vi "OE1022D_Operation_Continuous_or_Averaging.vi"() -> ()   [LabVIEW 2024]
uses:
  <vilib>/Utility/file.llb/Write Delimited Spreadsheet (string).vi
  <vilib>/Utility/file.llb/Write Delimited Spreadsheet (DBL).vi
  <vilib>/Analysis/NI_AALBase.lvlib
panel:
  in  "Add file info to file save":bool=TRUE
  in  "B Sensitivity":u16(ring)=20 items=["1 nV/fA", "2 nV/fA", "5 nV/fA", "10 nV/fA", "20 nV/fA", "50 nV/fA", "100 nV/fA", "200 nV/fA", "500 nV/fA", "1 uV/pA", "2 uV/pA", "5 uV/pA", "10 uV/pA", "20 uV/pA", "50 uV/pA", "100 uV/pA", "200 uV/pA", "500 uV/pA", "1 mV/nA", "2 mV/nA", "5 mV/nA", "10 mV/nA", "20 mV/nA", "50 mV/nA", "100 mV/nA", "200 mV/nA", "500 mV/nA", "1 V/uA"]
  out "Channel B Waveform Chart":dbl(graph)
  in  "Channel B Waveform Display":string(combo)="B-R"
  in  "Channel A Waveform Display":string(combo)="A-R"
  in  "A Sensitivity":u16(ring)=20 items=["1 nV/fA", "2 nV/fA", "5 nV/fA", "10 nV/fA", "20 nV/fA", "50 nV/fA", "100 nV/fA", "200 nV/fA", "500 nV/fA", "1 uV/pA", "2 uV/pA", "5 uV/pA", "10 uV/pA", "20 uV/pA", "50 uV/pA", "100 uV/pA", "200 uV/pA", "500 uV/pA", "1 mV/nA", "2 mV/nA", "5 mV/nA", "10 mV/nA", "20 mV/nA", "50 mV/nA", "100 mV/nA", "200 mV/nA", "500 mV/nA", "1 V/uA"]
  in  "File Path":path=path "C:/Users/Public/OneDrive/Desktop/test.txt"
  in  "Data Points":i32
  out "Channel AWaveform Chart":dbl(graph)
  out "θh1 (°) 2":sgl caption="θh1 (deg)" format="%.2f"
  out "Rh1 2":sgl caption="Rh1 (Vrms)" format="%.3p"
  out "Yh1 2":sgl caption="Yh1 (Vrms)" format="%.3p"
  out "Xh1 2":sgl caption="Xh1 (Vrms)" format="%.3p"
  out "Xh2 2":sgl caption="Xh2 (Vrms)" format="%.3p"
  out "Yh2 2":sgl caption="Yh2 (Vrms)" format="%.3p"
  out "Rh2 2":sgl caption="Rh2 (Vrms)" format="%.3p"
  out "噪声 2":sgl caption="Noise(Vrms)" format="%.3p"
  out "频率 (Hz) 2":sgl caption="Freq (Hz)" format="%#.3f"
  out "θ (°) 2":sgl caption="θ (deg)" format="%.2f"
  out "R 2":sgl caption="R (Vrms)" format="%.3p"
  out "Y 2":sgl caption="Y (Vrms)" format="%.3p"
  out "θh2 (°) 2":sgl caption="θh2 (deg)" format="%.2f"
  out "X 2":sgl caption="X (Vrms)" format="%.3p"
  out "Yh1":sgl caption="Yh1 (Vrms)" format="%.3p"
  out "Xh1":sgl caption="Xh1 (Vrms)" format="%.3p"
  out "θh2 (°)":sgl caption="θh2 (deg)" format="%.2f"
  out "Yh2":sgl caption="Yh2 (Vrms)" format="%.3p"
  out "Xh2":sgl caption="Xh2 (Vrms)" format="%.3p"
  out "Rh2":sgl caption="Rh2 (Vrms)" format="%.3p"
  out "θh1 (°)":sgl caption="θh1 (deg)" format="%.2f"
  out "Rh1":sgl caption="Rh1 (Vrms)" format="%.3p"
  out "噪声":sgl caption="Noise(Vrms)" format="%.3p"
  out "频率 (Hz)":sgl caption="Freq (Hz)" format="%#.3f"
  out "θ (°)":sgl caption="θ (deg)" format="%.2f"
  out "Y":sgl caption="Y (Vrms)" format="%.3p"
  out "X":sgl caption="X (Vrms)" format="%.3p"
  out "R":sgl caption="R (Vrms)" format="%.3p"
  out "AUX-ADC2 (V)":sgl format="%.3f"
  out "AUX-ADC1 (V)":sgl format="%.3f"
  out "AUX-ADC3 (V)":sgl format="%.3f"
  out "AUX-ADC4 (V)":sgl format="%.3f"
  out "错误输出":errorcluster
  out "序列号":string
  in  "OE1022D":refnum<visa-resource-name>="COM6"
  # "input 0 for continous"
  # "Choose the value to display on the graph. This is the quantity that is saved"
  # "Channel A"
  # "Channel B"
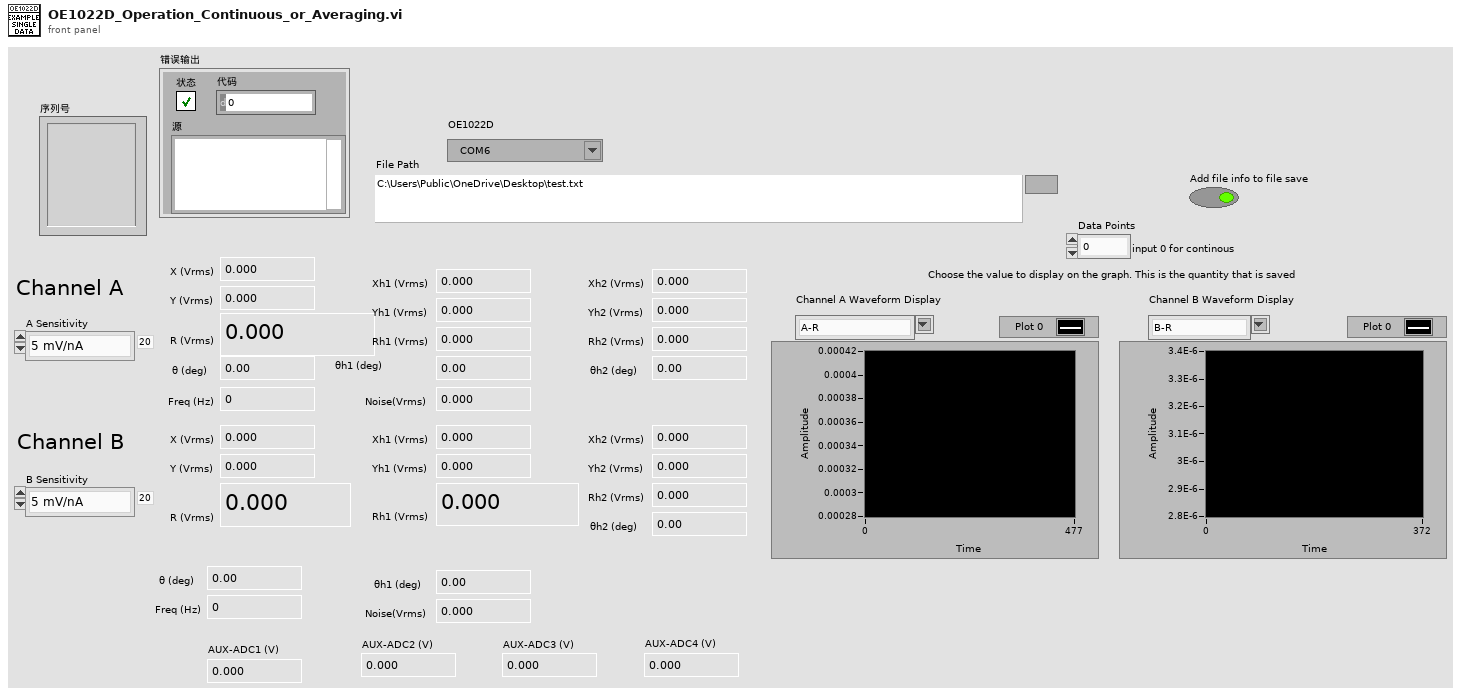
[diagram p1: front panel]
types:
  T1 = cluster{"AD1":dbl[], "AD2":dbl[], "AD3":dbl[], "AD4":dbl[]}
  T2 = cluster{"XB":dbl[], "YB":dbl[], "FrequencyB":dbl[], "NoiseB":dbl[], "Xh1B":dbl[], "Yh1B":dbl[], "Xh2B":dbl[], "Yh2B":dbl[], "Xh2B":dbl[]}
  T3 = cluster{"XA":dbl[], "YA":dbl[], "FrequencyA":dbl[], "NoiseA":dbl[], "Xh1A":dbl[], "Yh1A":dbl[], "Xh2A":dbl[], "Yh2A":dbl[]}
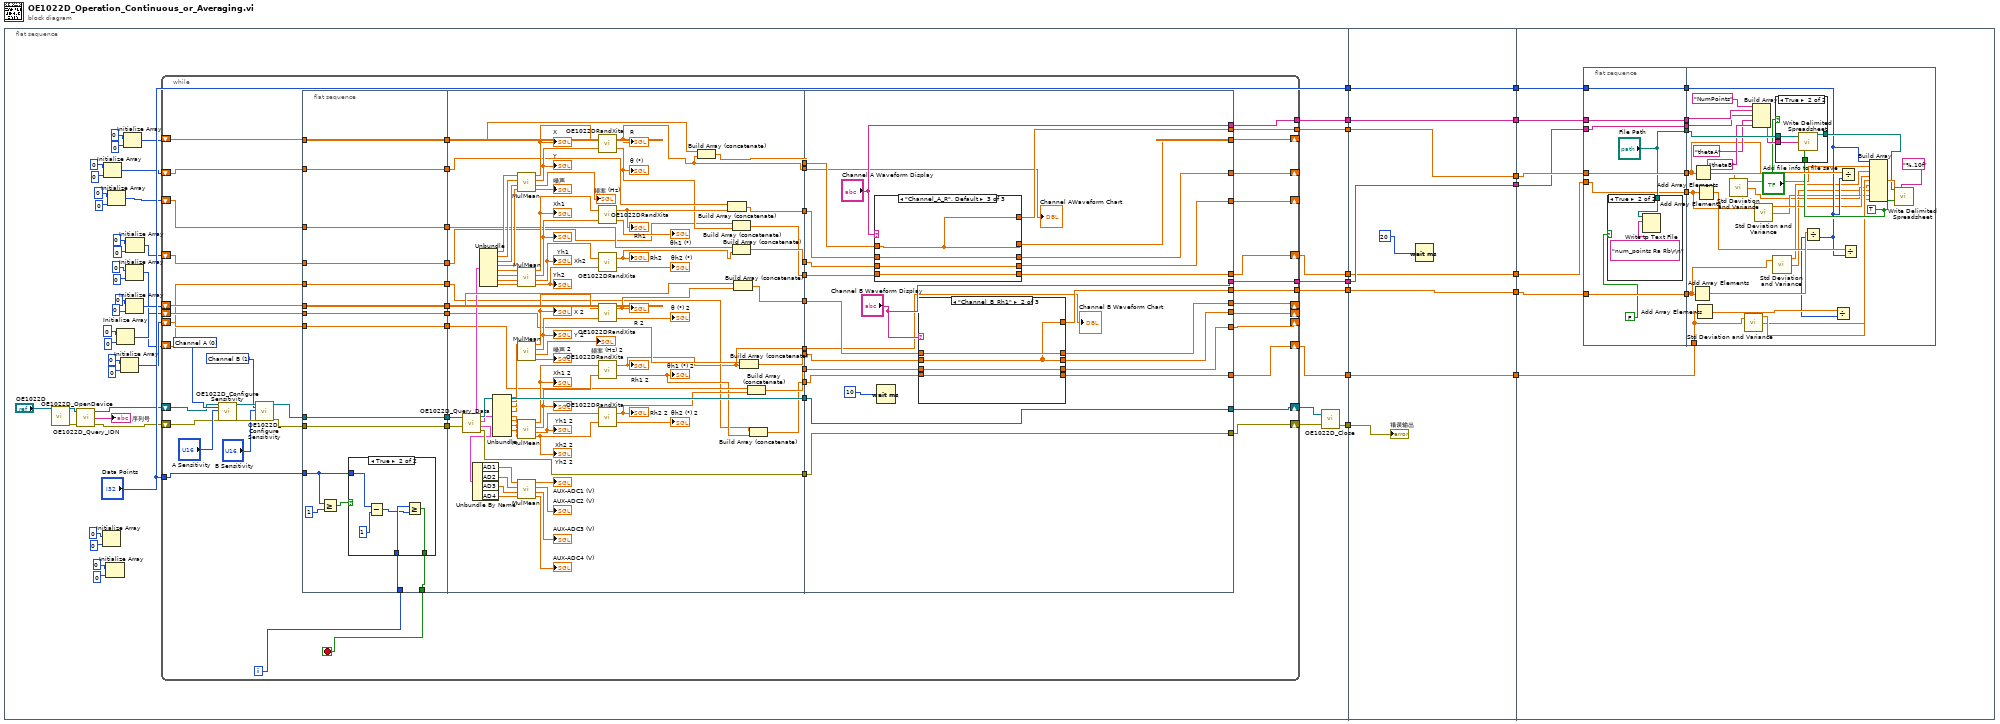
[diagram p0: block diagram]
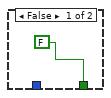
[diagram p2: hidden frame]
diagram:
  n1 = flat-sequence {
    tunnel: [w36] -> w15
    tunnel: [w35] -> w13
    tunnel: ["Data Points"] -> w11
    tunnel: [w30] -> w9
    tunnel: [w34] -> w7
    tunnel: [w33] -> w6
    tunnel: [w20] -> w3
    tunnel: [w21] -> w2
    tunnel: w15 -> [w270]
    tunnel: [w270] -> w14
    tunnel: w13 -> [w269]
    tunnel: [w269] -> w12
    tunnel: w11 -> [w268]
    tunnel: [w268] -> w10
    tunnel: w9 -> [w266]
    tunnel: [w265] -> w8
    tunnel: w7 -> [w265]
    tunnel: w6 -> [w264]
    tunnel: [w264] -> w5
    tunnel: [w263] -> w4
    tunnel: w3 -> [w263]
    tunnel: w2 -> [w262]
    tunnel: [w262] -> w1
    tunnel: w14 -> [w280]
    tunnel: w12 -> [w279]
    tunnel: w10 -> [w278]
    tunnel: w8 -> [w276]
    tunnel: w5 -> [w275]
    tunnel: w4 -> [w273]
    tunnel: w1 -> [w271]
    frame #0 {
      n2 = call "OE1022D_OpenDevice.vi"("VISA resource name"="OE1022D") -> ("VISA资源名称输出"=w58:refnum<visa-resource-name>, "错误输出"=w57:errorcluster)  [unwired: 17 in]
      n3 = call "OE1022D_Query_IDN.vi"("错误输入（无错误）"=w57, "VISA resource name"=w58) -> ("错误输出"=w28:errorcluster, "序列号"=→"序列号":string, "VISA resource name out"=w29:refnum<visa-resource-name>)  [unwired: 1 in]
      n4 = Initialize Array(0, 0) -> ()  [unwired: 1 out]
      n5 = Initialize Array(0, 0) -> (w43:i32[])
      n6 = Initialize Array(0, 0) -> ()  [unwired: 1 out]
      n7 = Initialize Array(0, 0) -> (w44:i32[])
      n8 = Initialize Array(0, 0) -> (w37:i32[])
      n9 = Initialize Array(0, 0) -> (w38:i32[])
      n10 = Initialize Array(0, 0) -> (w54:i32[])
      n11 = Initialize Array(0, 0) -> (w22:i32[])
      n12 = Initialize Array(0, 0) -> (w49:i32[])
      n13 = Initialize Array(0, 0) -> (w23:i32[])
      n14 = while {
        shift-right: [w113] -> _
        shift-left: w54 -> [w112]
        shift-right: [w110] -> _
        shift-left: w49 -> [w109]
        tunnel: "Data Points" -> [w102]
        shift-right: [w90] -> _
        shift-left: w43 -> [w92]
        shift-right: [w86] -> _
        shift-left: w44 -> [w89]
        shift-right: [w79] -> _
        shift-left: w37 -> [w85]
        shift-right: [w78] -> _
        shift-left: w38 -> [w84]
        tunnel: [w77] -> w36
        tunnel: [w76] -> w35
        tunnel: [w75] -> w34
        tunnel: [w74] -> w33
        shift-right: [w73] -> w32
        shift-left: w28 -> [w70]
        shift-right: [w72] -> w31
        shift-left: w29 -> [w71]
        shift-right: [w62] -> w20
        shift-left: w23 -> [w66]
        shift-right: [w63] -> w21
        shift-left: w22 -> [w64]
        i -> [w104]
        stop <- w103 stop-if-true
        w95 = u8 1 items=["Channel A", "Channel B"] ("OE1022D A/B")
        w101 = u8 0 items=["Channel A", "Channel B"] ("OE1022D A/B")
        n15 = call "OE1022D_Configure Sensitivity.vi"("VISA resource name"=w71, "OE1022D A/B"=w101, "Sensitivity"="A Sensitivity", "error in (no error)"=w70) -> ("VISA resource name out"=w96:refnum<visa-resource-name>, "error out"=w97:errorcluster)  [unwired: 14 in]
        n16 = call "OE1022D_Configure Sensitivity.vi"("VISA resource name"=w96, "OE1022D A/B"=w95, "Sensitivity"="B Sensitivity", "error in (no error)"=w97) -> ("VISA resource name out"=w99:refnum<visa-resource-name>, "error out"=w98:errorcluster)  [unwired: 14 in]
        n17 = flat-sequence {
          tunnel: w109 -> [w128]
          tunnel: w112 -> [w129]
          tunnel: w99 -> [w130]
          tunnel: w98 -> [w131]
          tunnel: [w131] -> w108
          tunnel: [w130] -> w107
          tunnel: [w129] -> w106
          tunnel: [w128] -> w105
          tunnel: w104 -> [w127]
          tunnel: [w126] -> w103
          tunnel: w102 -> [w124]
          tunnel: [w122] -> w93
          tunnel: w92 -> [w122]
          tunnel: w89 -> [w121]
          tunnel: [w121] -> w88
          tunnel: w85 -> [w120]
          tunnel: w84 -> [w119]
          tunnel: [w120] -> w83
          tunnel: [w119] -> w82
          tunnel: [w118] -> w67
          tunnel: w66 -> [w118]
          tunnel: [w117] -> w65
          tunnel: w64 -> [w117]
          tunnel: [w210] -> w116
          tunnel: [w209] -> w115
          tunnel: [w161] -> w114
          tunnel: [w157] -> w111
          tunnel: w108 -> [w212]
          tunnel: w107 -> [w211]
          tunnel: w106 -> [w162]
          tunnel: w105 -> [w159]
          tunnel: w93 -> [w155]
          tunnel: [w154] -> w91
          tunnel: w88 -> [w152]
          tunnel: [w151] -> w87
          tunnel: w83 -> [w148]
          tunnel: w82 -> [w149]
          tunnel: [w147] -> w81
          tunnel: [w146] -> w80
          tunnel: [w142] -> w69
          tunnel: [w144] -> w68
          tunnel: w67 -> [w141]
          tunnel: w65 -> [w140]
          tunnel: [w139] -> w61
          tunnel: [w138] -> w60
          tunnel: w116 -> [w235]
          tunnel: w115 -> [w236]
          tunnel: w114 -> [w234]
          tunnel: [w232] -> w113
          tunnel: w111 -> [w228]
          tunnel: [w227] -> w110
          tunnel: [w236] -> w72
          tunnel: [w235] -> w73
          tunnel: w91 -> [w233]
          tunnel: [w231] -> w90
          tunnel: w87 -> [w230]
          tunnel: [w229] -> w86
          tunnel: w81 -> [w223]
          tunnel: w80 -> [w226]
          tunnel: [w225] -> w79
          tunnel: [w224] -> w78
          tunnel: [w222] -> w77
          tunnel: [w221] -> w76
          tunnel: ["Channel A Waveform Display"] -> w75
          tunnel: ["Channel B Waveform Display"] -> w74
          tunnel: w69 -> [w217]
          tunnel: [w216] -> w62
          tunnel: [w215] -> w63
          tunnel: w68 -> [w218]
          tunnel: w61 -> [w214]
          tunnel: w60 -> [w213]
          frame #0 {
            n18 = Greater Or Equal?(x=w124, y=1) -> (x >= y?=w123:bool)
            n19 = case shown="True" w123 {
              tunnel: w127 -> [_ w137]
              tunnel: [FALSE w136] -> w126
              tunnel: w124 -> [_ w133]
              frame False {
              }
              frame True {
                n20 = Subtract(x=w133, y=1) -> (x-y=w134:i32)
                n21 = Greater Or Equal?(x=w137, y=w134) -> (x >= y?=w136:bool)
              }
            }
          }
          frame #1 {
            n22 = call "OE1022D_Query_Data.vi"("错误输入（无错误）"=w212, "VISA resource name"=w211) -> ("error out"=w210:errorcluster, "输出簇ADC"=w164:T1, "输出簇B"=w163:T2, "VISA resource name out"=w209:refnum<visa-resource-name>, "输出簇A"=w158:T3)  [unwired: 3 in]
            n23 = Unbundle By Name(w164) -> ("AD1"=w205:dbl[], "AD2"=w206:dbl[], "AD3"=w207:dbl[], "AD4"=w208:dbl[])
            n24 = Unbundle(w158) -> ("XA"=w169:dbl[], "YA"=w170:dbl[], "FrequencyA"=w171:dbl[], "NoiseA"=w172:dbl[], "Xh1A"=w177:dbl[], "Yh1A"=w178:dbl[], "Xh2A"=w179:dbl[], "Yh2A"=w180:dbl[])
            n25 = Unbundle(w163) -> ("XB"=w194:dbl[], "YB"=w193:dbl[], "FrequencyB"=w192:dbl[], "NoiseB"=w191:dbl[], "Xh1B"=w190:dbl[], "Yh1B"=w189:dbl[], "Xh2B"=w188:dbl[], "Yh2B"=w187:dbl[])  [unwired: 1 out]
            n26 = call "MulMean.vi"("IN 4"=w172, "IN 3"=w171, "IN 2"=w170, "IN 1"=w169) -> ("mean 4"=→"噪声":dbl, "mean 3"=→"频率 (Hz)":dbl, "mean 2"=w175:dbl, "mean 1"=w174:dbl)  [unwired: 4 in]
            "X" <- w174
            "Y" <- w175
            n27 = call "MulMean.vi"("IN 4"=w180, "IN 3"=w179, "IN 2"=w178, "IN 1"=w177) -> ("mean 4"=w185:dbl, "mean 3"=w184:dbl, "mean 2"=w182:dbl, "mean 1"=w181:dbl)  [unwired: 4 in]
            "Xh2" <- w184
            "Yh2" <- w185
            "Xh1" <- w181
            "Yh1" <- w182
            n28 = call "MulMean.vi"("IN 4"=w191, "IN 3"=w192, "IN 2"=w193, "IN 1"=w194) -> ("mean 4"=→"噪声 2":dbl, "mean 3"=→"频率 (Hz) 2":dbl, "mean 2"=w199:dbl, "mean 1"=w198:dbl)  [unwired: 4 in]
            "X 2" <- w198
            "Y 2" <- w199
            n29 = call "MulMean.vi"("IN 4"=w187, "IN 3"=w188, "IN 2"=w189, "IN 1"=w190) -> ("mean 4"=w203:dbl, "mean 3"=w202:dbl, "mean 2"=w201:dbl, "mean 1"=w200:dbl)  [unwired: 4 in]
            "Yh2 2" <- w203
            "Xh2 2" <- w202
            "Xh1 2" <- w200
            "Yh1 2" <- w201
            n30 = call "MulMean.vi"("IN 4"=w208, "IN 3"=w207, "IN 2"=w206, "IN 1"=w205) -> ("mean 4"=→"AUX-ADC4 (V)":dbl, "mean 3"=→"AUX-ADC3 (V)":dbl, "mean 2"=→"AUX-ADC2 (V)":dbl, "mean 1"=→"AUX-ADC1 (V)":dbl)  [unwired: 4 in]
            n31 = call "OE1022DRandXita.vi"("Y"=w175, "X"=w174) -> ("θ (°)"=w143:dbl, "R"=w138:dbl)
            "R" <- w138
            "θ (°)" <- w143
            n32 = call "OE1022DRandXita.vi"("Y"=w182, "X"=w181) -> ("θ (°)"=→"θh1 (°)":dbl, "R"=w156:dbl)
            "Rh1" <- w156
            n33 = call "OE1022DRandXita.vi"("Y"=w185, "X"=w184) -> ("θ (°)"=→"θh2 (°)":dbl, "R"=w153:dbl)
            "Rh2" <- w153
            n34 = call "OE1022DRandXita.vi"("Y"=w199, "X"=w198) -> ("θ (°)"=→"θ (°) 2":dbl, "R"=w160:dbl)
            "R 2" <- w160
            n35 = call "OE1022DRandXita.vi"("Y"=w201, "X"=w200) -> ("θ (°)"=w145:dbl, "R"=w139:dbl)
            "Rh1 2" <- w139
            "θh1 (°) 2" <- w145
            n36 = call "OE1022DRandXita.vi"("Y"=w203, "X"=w202) -> ("θ (°)"=→"θh2 (°) 2":dbl, "R"=w150:dbl)
            "Rh2 2" <- w150
            n37 = Build Array (concatenate)(w162, w138) -> (w161:dbl[])
            n38 = Build Array (concatenate)(w155, w156) -> (w154:dbl[])
            n39 = Build Array (concatenate)(w141, w143) -> (w142:dbl[])
            n40 = Build Array (concatenate)(w152, w153) -> (w151:dbl[])
            n41 = Build Array (concatenate)(w159, w160) -> (w157:dbl[])
            n42 = Build Array (concatenate)(w148, w139) -> (w147:dbl[])
            n43 = Build Array (concatenate)(w149, w150) -> (w146:dbl[])
            n44 = Build Array (concatenate)(w140, w145) -> (w144:dbl[])
          }
          frame #2 {
            n45 = case shown="\"Channel_A_R\", Default" "Channel A Waveform Display" {
              tunnel: w234 -> [w253 w257 w259]
              tunnel: [w253 w257 w259] -> w232
              tunnel: w233 -> [w251 w256 w261]
              tunnel: [w251 w256 w261] -> w231
              tunnel: w230 -> [w252 w255 w260]
              tunnel: [w252 w255 w260] -> w229
              tunnel: [w251 w255 w259] -> w222
              tunnel: w217 -> [w250 w254 w258]
              tunnel: [w250 w254 w258] -> w216
              frame "Channel_A_Rh1" {
              }
              frame "Channel_A_Rh2" {
              }
              frame "Channel_A_R", Default {
              }
            }
            n46 = Wait (ms)(milliseconds to wait=10) -> ()  [unwired: 1 out]
            n47 = case shown="\"Channel_B_Rh1\"" "Channel B Waveform Display" {
              tunnel: [w241 w243 w247] -> w221
              tunnel: w228 -> [w241 w245 w249]
              tunnel: [w241 w245 w249] -> w227
              tunnel: w226 -> [w240 w244 w247]
              tunnel: [w240 w244 w247] -> w224
              tunnel: [w239 w243 w248] -> w225
              tunnel: w223 -> [w239 w243 w248]
              tunnel: w218 -> [w238 w242 w246]
              tunnel: [w238 w242 w246] -> w215
              frame "Channel_B_R", Default {
              }
              frame "Channel_B_Rh1" {
              }
              frame "Channel_B_Rh2" {
              }
            }
            "Channel AWaveform Chart" <- w213
            "Channel B Waveform Chart" <- w214
          }
        }
      }
      n48 = call "OE1022D_Close.vi"("错误输入（无错误）"=w32, "VISA resource name"=w31) -> ("错误输出"=w30:errorcluster)  [unwired: 1 in]
    }
    frame #1 {
      n49 = Wait (ms)(milliseconds to wait=20) -> ()  [unwired: 1 out]
      "错误输出" <- w266
    }
    frame #2 {
      n50 = flat-sequence {
        tunnel: w278 -> [w290]
        tunnel: w279 -> [w291]
        tunnel: w280 -> [w292]
        tunnel: [w292] -> w284
        tunnel: [w291] -> w283
        tunnel: [w290] -> w282
        tunnel: ["File Path"] -> w281
        tunnel: [w287] -> w277
        tunnel: w276 -> [w287]
        tunnel: w275 -> [w286]
        tunnel: [w286] -> w274
        tunnel: w273 -> [w285]
        tunnel: [w285] -> w272
        tunnel: w284 -> [w303]
        tunnel: w283 -> [w306]
        tunnel: w282 -> [w310]
        tunnel: w281 -> [w318]
        tunnel: w277 -> [w316]
        tunnel: w274 -> [w315]
        tunnel: w272 -> [w304]
        tunnel: w271 -> [w305]
        frame #0 {
          n51 = case shown="True" FALSE {
            tunnel: "File Path" -> [_ w294]
            frame False {
            }
            frame True {
              n52 = Write to Text File(file (use dialog)=w294, text="num_points Ra Rb\r\n") -> ()  [unwired: 2 in, 3 out]
            }
          }
        }
        frame #1 {
          w317 = TRUE
          n53 = Add Array Elements(numeric array=w306) -> (sum=w320:dbl)
          n54 = Add Array Elements(numeric array=w303) -> (sum=w322:dbl)
          n55 = Add Array Elements(numeric array=w305) -> (sum=w311:dbl)
          n56 = Add Array Elements(numeric array=w304) -> (sum=w312:dbl)
          n57 = call <vilib>:"Std Deviation and Variance.vi"("X"=w303) -> ("mean"=w302:dbl, "standard deviation"=w296:dbl)  [unwired: 1 in, 1 out]
          n58 = call <vilib>:"Std Deviation and Variance.vi"("X"=w305) -> ("mean"=w299:dbl, "standard deviation"=w298:dbl)  [unwired: 1 in, 1 out]
          n59 = Build Array("NumPoints", w316, w315, "thetaA", "thetaB") -> (w313:string[])
          n60 = call <vilib>:"Std Deviation and Variance.vi"("X"=w304) -> ("mean"=w300:dbl, "standard deviation"=w297:dbl)  [unwired: 1 in, 1 out]
          n61 = call <vilib>:"Std Deviation and Variance.vi"("X"=w306) -> ("mean"=w301:dbl, "standard deviation"=w295:dbl)  [unwired: 1 in, 1 out]
          n62 = case shown="True" "Add file info to file save" {
            tunnel: [w324 w328] -> w319
            tunnel: w318 -> [w324 w327]
            tunnel: w317 -> [_ w326]
            tunnel: w313 -> [_ w325]
            frame False {
            }
            frame True {
              n63 = call-poly <vilib>:"Write Delimited Spreadsheet.vi"("file path (dialog if empty)"=w327, "1D data"=w325, "append to file? (new file:F)"=w326) -> ("new file path (Not A Path if cancelled)"=w328:path)  [unwired: 11 in, 1 out]
            }
          }
          n64 = Divide(x=w320, y=w310) -> ()  [unwired: 1 out]
          n65 = Divide(x=w311, y=w310) -> ()  [unwired: 1 out]
          n66 = Divide(x=w322, y=w310) -> ()  [unwired: 1 out]
          n67 = Divide(x=w312, y=w310) -> ()  [unwired: 1 out]
          n68 = Build Array(w310, w302, w301, w300, w299, w296, w295, w297, w298) -> (w321:dbl[])
          n69 = call-poly <vilib>:"Write Delimited Spreadsheet.vi"("file path (dialog if empty)"=w319, "format (%.3f)"="%.10f", "1D data"=w321, "append to file? (new file:F)"=w317) -> ()  [unwired: 10 in, 2 out]
        }
      }
    }
  }
